vi "游程编码.vi"() -> ()   [LabVIEW 2020]
panel:
  out "输出编码：":cluster{"Value":i32, "Counter":i32}[](array[cluster])
  in  "输入序列：":i32[](array[numeric])=[0, 0, 1, 1, 0, 1, 0, 0, 0, 1, 0, 0, 1, 1]
  # "游程编码\n游程编码又称“运行长度编码”或“行程编码”，是一种统计编码，该编码属于无损压缩编码。对于二值图有效。 \n\n行程编码的基本原理是：用一个符号值或串长代替具有相同值的连续符号（连续符号构成了一段连续的“行程”。行程编码因此而得名），使符号长度少于原始数据的长度。例如：5555557777733322221111111行程编码为：（5，6）（7，5）（3，3）（2，4）（l，7）。可见，行程编码的位数远远少于原始字符串的位数。并不是所有的行程编码都远远少于原始字符串的位数，但行程编码也成为了一种压缩工具。例如：555555是6个字符而（5，6）是5个字符，这也存在压缩量的问题，自然也会出现其他方式的压缩工具。\n\n在对图像数据进行编码时，沿一定方向排列的具有相同灰度值的像素可看成是连续符号，用字串代替这些连续符号，可大幅度减少数据量。\n行程编码分为定长行程编码和不定长行程编码两种类型。行程编码是连续精确的编码，在传输过程中，如果其中一位符号发生错误，即可影响整个编码序列，使行程编码无法还原回原始数据。\n\n操作：\n1) 改变数组序列中的数据值；\n2)运行程序后，输出数组输出“值”和“行程”"
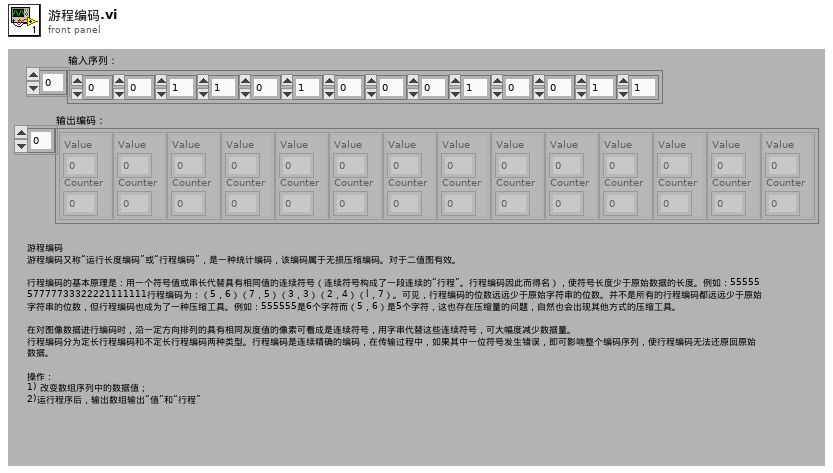
[diagram p1: front panel]
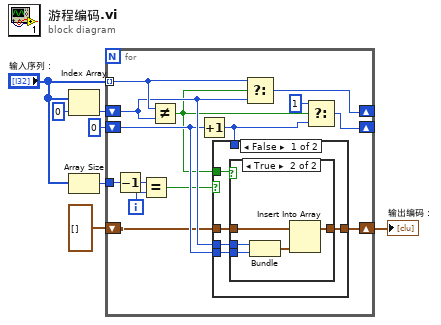
[diagram p0: block diagram]
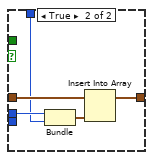
[diagram p3: hidden frame]
diagram:
  n1 = Index Array(array="输入序列：", index=0) -> (element=w5:i32)
  n2 = Array Size(array="输入序列：") -> (size(s)=w1:i32)
  n3 = for {
    shift-right: [w21] -> _
    shift-left: w5 -> [w14]
    shift-right: [w20] -> _
    shift-left: 0 ("index") -> [w13]
    tunnel: "输入序列：" -> [w15] mode=indexing
    shift-right: [w9] -> w4
    shift-left: cluster{"Numeric":i32, "index":i32}[] [] -> [w12]
    tunnel: w1 -> [w19]
    i -> [w16]
    n4 = Decrement(x=w19) -> (x-1=w17:i32)
    n5 = Equal?(x=w17, y=w16) -> (x = y?=w11:bool)
    n6 = Not Equal?(x=w15, y=w14) -> (x != y?=w10:bool)
    n7 = Increment(x=w13) -> (x+1=w8:i32)
    n8 = case shown="False" w11 {
      tunnel: w14 -> [w26 w35]
      tunnel: w13 -> [w25 _]
      tunnel: w12 -> [w24 w36]
      tunnel: w10 -> [w23 _]
      tunnel: [w22 w33] -> w9
      tunnel: w8 -> [_ w34]
      frame False {
        n9 = case shown="True" w23 {
          tunnel: w26 -> [_ w31]
          tunnel: w25 -> [_ w30]
          tunnel: w24 -> [w27 w29]
          tunnel: [w27 w28] -> w22
          frame False {
          }
          frame True {
            n10 = Bundle("Numeric"=w31, "index"=w30) -> (w32:cluster{"Numeric":i32, "index":i32})  [unwired: 1 out]
            n11 = Insert Into Array(array=w29, new element=w32) -> (w28:cluster{"Numeric":i32, "index":i32}[])  [unwired: 1 in]
          }
        }
      }
      frame True {
        n12 = Bundle("Numeric"=w35, w34) -> (w37:cluster{"Numeric":i32, i32})  [unwired: 1 out]
        n13 = Insert Into Array(array=w36, new element=w37) -> (w33:cluster{"Numeric":i32, "index":i32}[])  [unwired: 1 in]
      }
    }
    n14 = Select(t=w15, s=w10, f=w14) -> (s? t:f=w21:i32)
    n15 = Select(t=1 ("f"), s=w10, f=w8) -> (s? t:f=w20:i32)
  }
  "输出编码：" <- w4
